vi "TailInsertionBenchmark_LargeData.vi"() -> ()   [LabVIEW 2013]
uses:
  ImpSelectionEnum.ctl
  source/LapDog.Collections.Lists/ListImp/ListImp.lvclass
  source/LapDog.Collections.Lists.Implementations/BufferedArray/BufferedArray.lvclass
  source/LapDog.Collections.Lists/StringList/StringList.lvclass
panel:
  out "Elements Created":i32
  in  "Num of Elements":i32
  in  "Element Size (kB)":i32
  in  "Implementation":T1
  out "Buffered Array List Imp (ms)":u32
  out "Default List Imp (ms)":u32
  out "error out":errorcluster
  # "Large Data Tail Insertion"
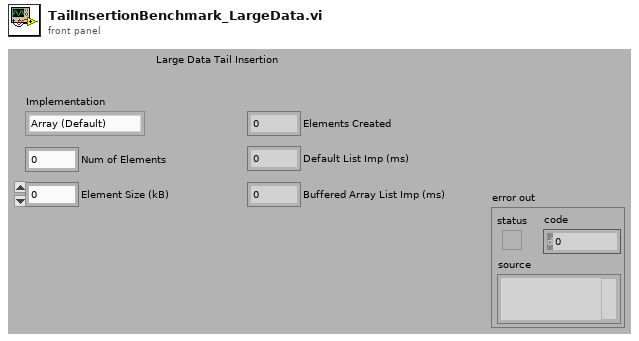
[diagram p1: front panel]
types:
  T1 = typedef "ImpSelectionEnum.ctl" = enum16{"Array (Default)", "Buffered Array"}
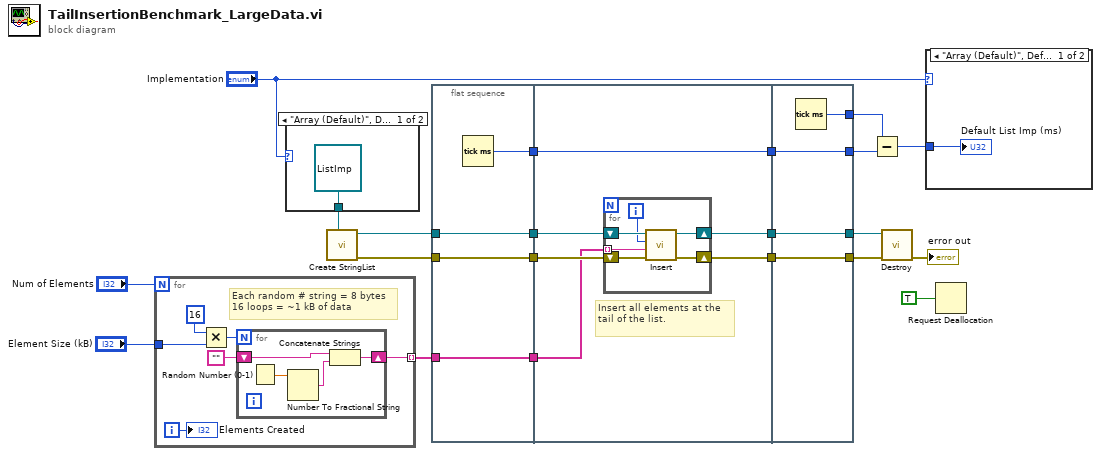
[diagram p0: block diagram]
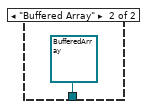
[diagram p2: hidden frame]
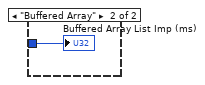
[diagram p3: hidden frame]
diagram:
  n1 = for {
    N: "Num of Elements" -> [_]
    tunnel: "Element Size (kB)" -> [w24]
    tunnel: [w23] -> w1 mode=indexing
    i -> [w22]
    # "Each random # string = 8 bytes\n16 loops = ~1 kB of data"
    n2 = Multiply(x=16, y=w24) -> (x*y=w25:i32)
    n3 = for {
      N: w25 -> [_]
      shift-right: [w29] -> w23
      shift-left: "" -> [w28]
      n4 = Random Number (0-1)() -> (number: 0 to 1=w31:dbl)
      n5 = Number To Fractional String(number=w31) -> (F-format string=w30:string)  [unwired: 3 in]
      n6 = Concatenate Strings(w28, w30) -> (w29:string)
    }
    "Elements Created" <- w22
  }
  n7 = case shown="\"Array (Default)\", Default" "Implementation" {
    tunnel: [refnum<class "ListImp.lvclass"> refnum ("LapDog.Collections.v0.Lists.lvlib:ListImp.lvclass") refnum<class "BufferedArray.lvclass"> refnum ("LapDog.Collections.v0.Lists.Implementations.lvlib:BufferedArray.lvclass")] -> w20
    frame "Array (Default)", Default {
    }
    frame "Buffered Array" {
    }
  }
  n8 = call "Create StringList.vi"("List Implementation (Array)"=w20) -> ("error out"=w16:errorcluster, "StringList out"=w18:refnum<class "StringList.lvclass">)  [unwired: 9 in]
  n9 = flat-sequence {
    tunnel: [w37] -> w21
    tunnel: [w36] -> w19
    tunnel: w18 -> [w36]
    tunnel: [w35] -> w17
    tunnel: w16 -> [w35]
    tunnel: [w34] -> w2
    tunnel: w1 -> [w34]
    tunnel: w21 -> [w39]
    tunnel: w19 -> [w43]
    tunnel: w17 -> [w42]
    tunnel: [w41] -> w15
    tunnel: [w40] -> w14
    tunnel: [w39] -> w13
    tunnel: w2 -> [w38]
    tunnel: [w52] -> w10
    tunnel: [w53] -> w9
    tunnel: w15 -> [w53]
    tunnel: w14 -> [w52]
    tunnel: w13 -> [w50]
    tunnel: [w51] -> w12
    tunnel: [w50] -> w11
    frame #0 {
      n10 = Tick Count (ms)() -> (millisecond timer value=w37:u32)
    }
    frame #1 {
      # "Insert all elements at the tail of the list."
      n11 = for {
        shift-right: [w48] -> w41
        shift-left: w43 -> [w49]
        shift-right: [w45] -> w40
        shift-left: w42 -> [w46]
        tunnel: w38 -> [w44] mode=indexing
        i -> [w47]
        n12 = call-dynamic "Insert.vi"("error in (no error)"=w46, "String"=w44, "Index"=w47, "StringList in"=w49) -> ("error out"=w45:errorcluster, "StringList out"=w48:refnum<class "StringList.lvclass">)  [unwired: 6 in]
      }
    }
    frame #2 {
      n13 = Tick Count (ms)() -> (millisecond timer value=w51:u32)
    }
  }
  n14 = Subtract(x=w12, y=w11) -> (x-y=w7:u32)
  n15 = call-dynamic "Destroy.vi"("error in (no error)"=w10, "StringList in"=w9) -> ("error out"=→"error out":errorcluster)  [unwired: 9 in]
  n16 = case shown="\"Array (Default)\", Default" "Implementation" {
    tunnel: w7 -> [w54 w55]
    frame "Array (Default)", Default {
      "Default List Imp (ms)" <- w54
    }
    frame "Buffered Array" {
      "Buffered Array List Imp (ms)" <- w55
    }
  }
  n17 = Request Deallocation(TRUE ("flag")) -> ()
